vi "CSM Example - Caller is NOT a CSM.vi"() -> ()   [LabVIEW 2017]
uses:
  user.lib/_NEVSTOP/Communicable State Machine(CSM)/_Support/Common/Format Timestamp.vi
  user.lib/_NEVSTOP/Communicable State Machine(CSM)/Communicable State Machine.lvlib
  1. Create a reuse Module/1. Create a reuse Module.lvlib
panel:
  in  "UI: Front Panel State >> Close":bool
  in  "UI: Front Panel State >> Open":bool
  in  "API: Get Level":bool
  in  "Selected Module":string(combo)="SubModule0"
  in  "Level":dbl min=0.0 max=1.0 step=0.1
  out "Status History":string
  in  "API: Stop":bool
  in  "API: Start":bool
  in  "Unregister Status Change":bool
  in  "Register Status Change":bool
  out "error":errorcluster
  in  "Stop Module":bool
  in  "Start Module":bool
  out "Exist?":bool
  # "#CSM-Example Overview\n\n1. The purpose of this example is to demonstrate how to invoke the CSM module from other framework application. In this scenario, inter-module communication solely relies on Post/Send Message API and module status change user event. \n\nThis example asynchronously calls two instances of \"CSM Reuse Module.vi\", providing dynamic subscription to messages and manipulation of the underlying Module through the API."
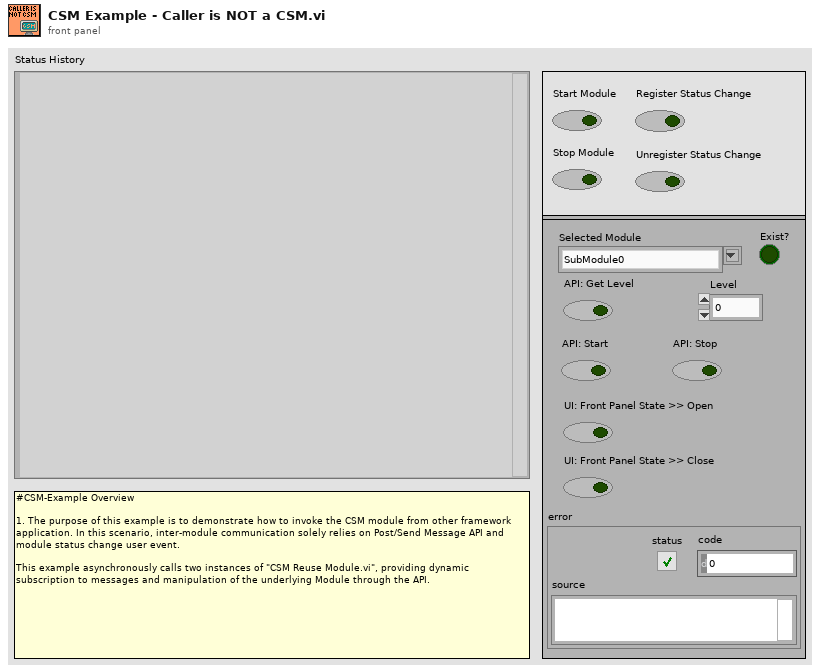
[diagram p1: front panel]
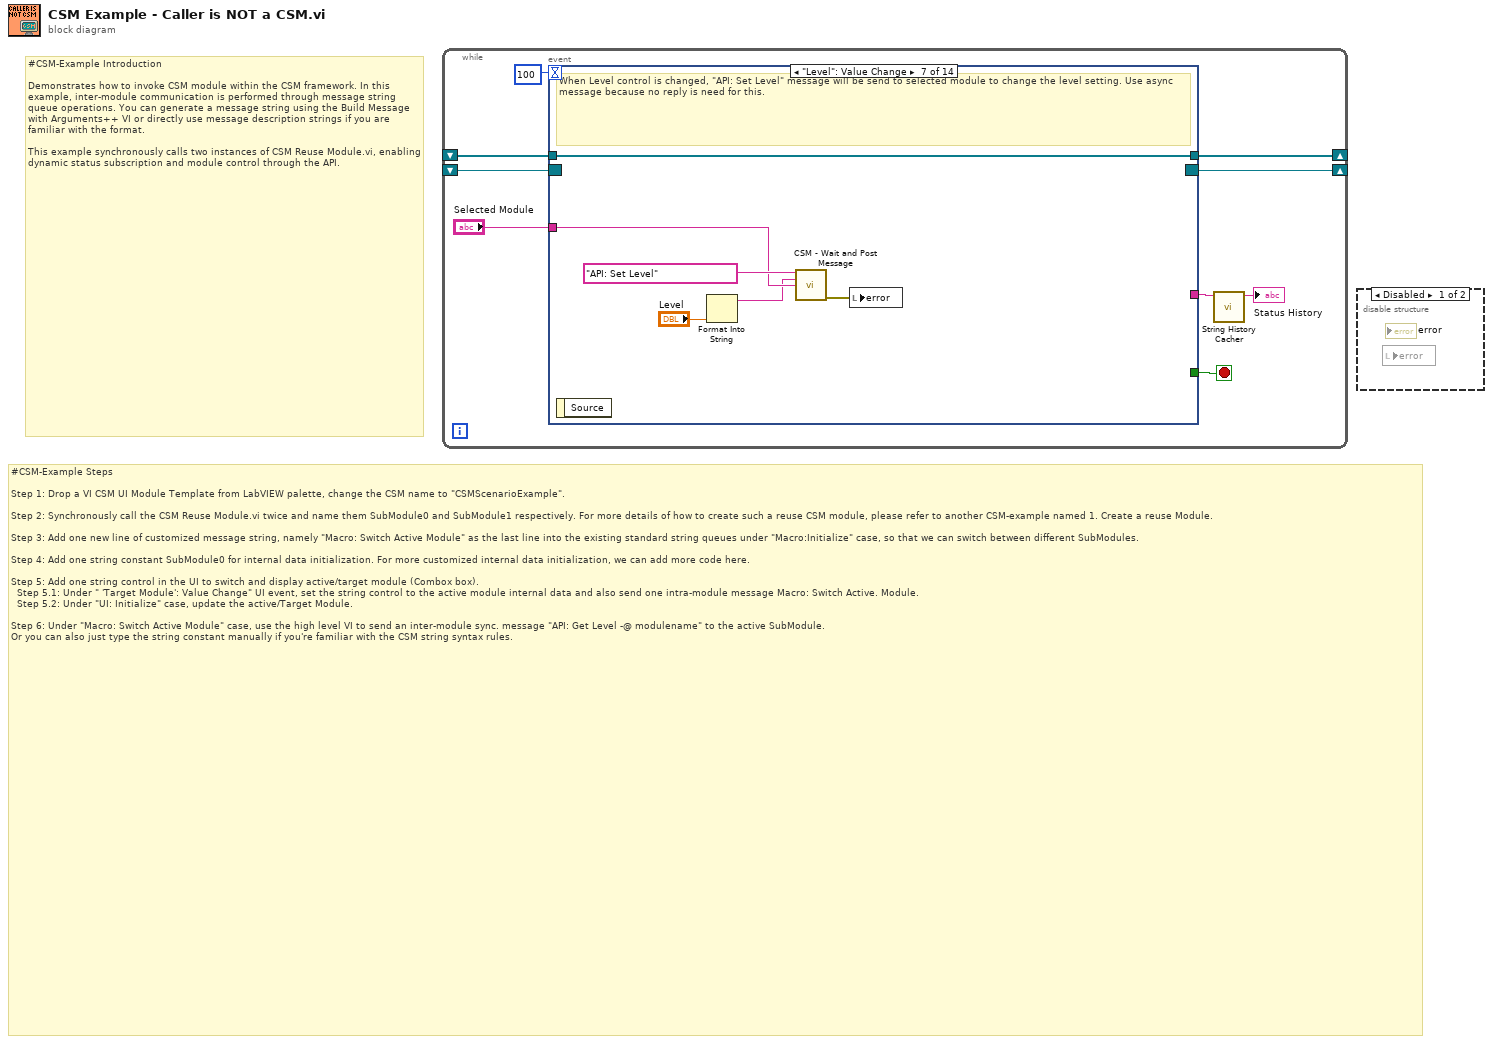
[diagram p0: block diagram]
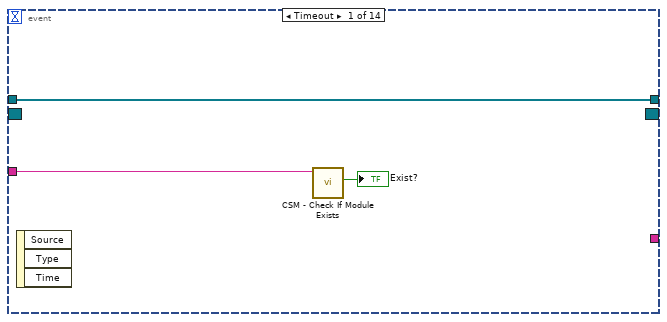
[diagram p3: hidden frame]
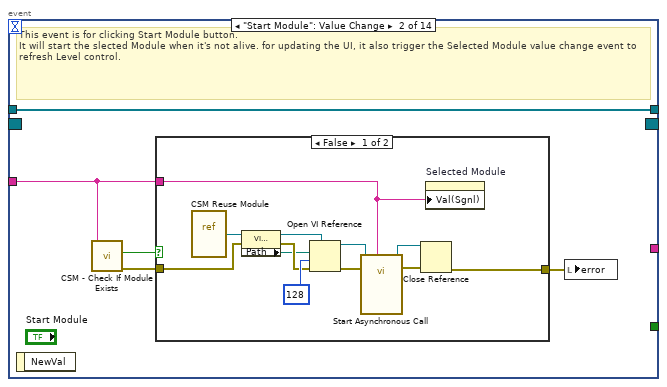
[diagram p4: hidden frame]
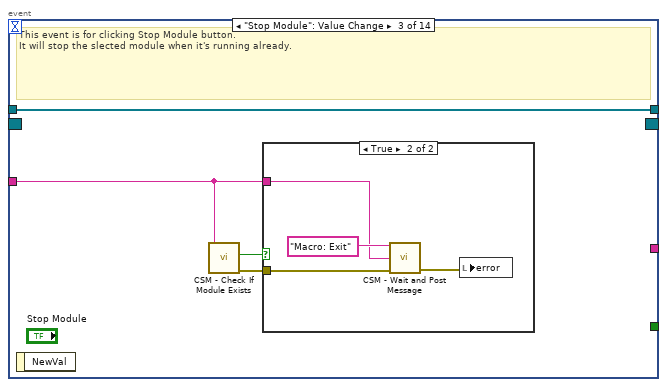
[diagram p6: hidden frame]
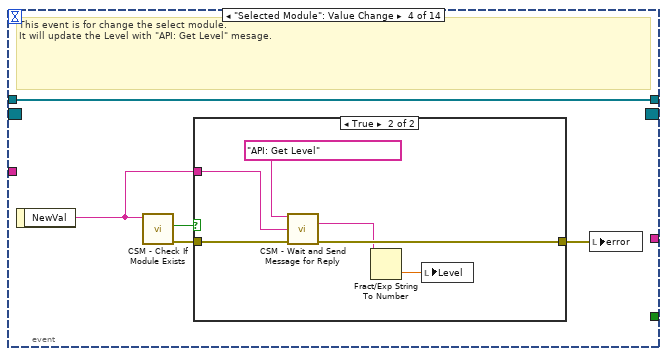
[diagram p8: hidden frame]
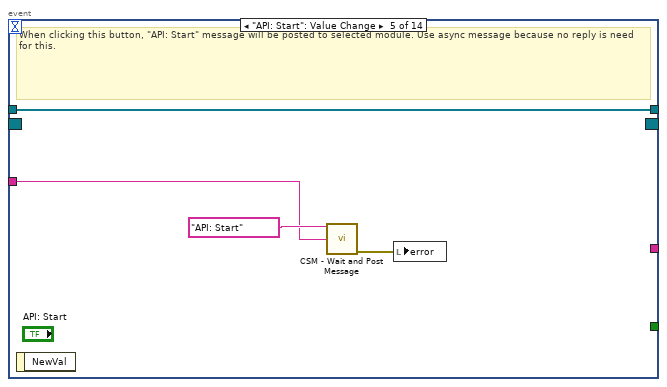
[diagram p10: hidden frame]
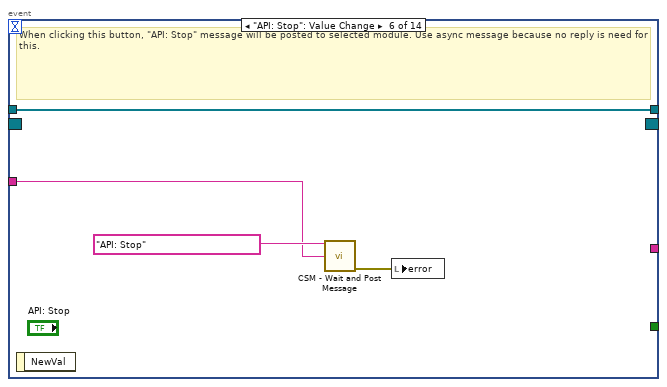
[diagram p11: hidden frame]
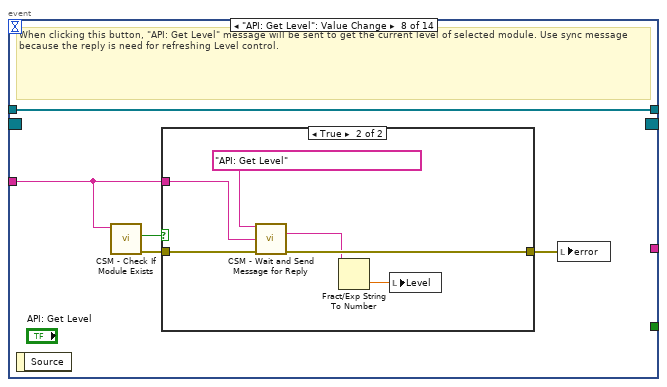
[diagram p12: hidden frame]
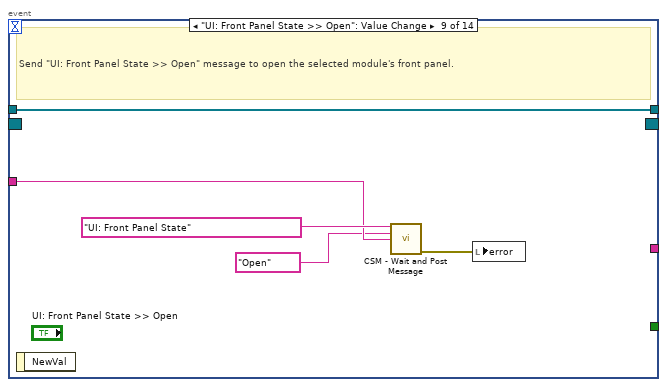
[diagram p14: hidden frame]
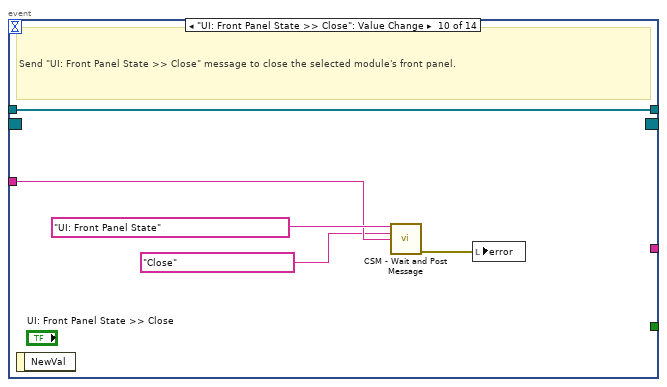
[diagram p15: hidden frame]
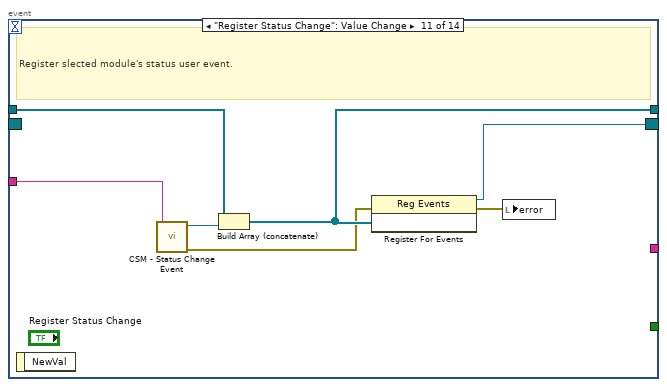
[diagram p16: hidden frame]
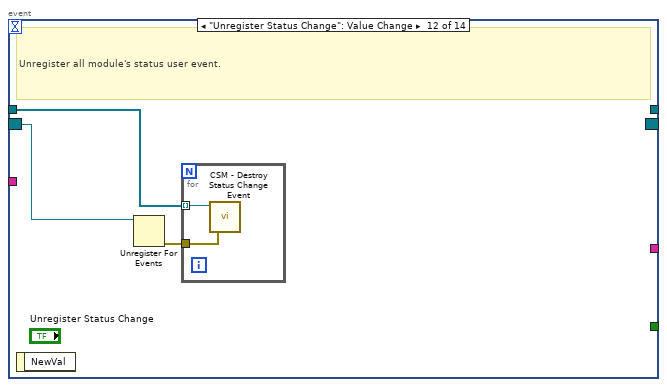
[diagram p17: hidden frame]
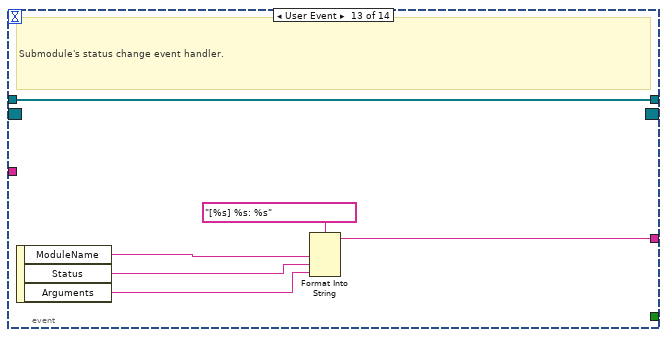
[diagram p18: hidden frame]
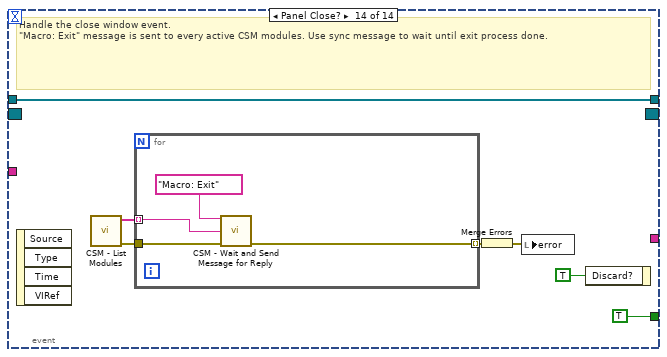
[diagram p19: hidden frame]
diagram:
  # "#CSM-Example Steps\n\nStep 1: Drop a VI CSM UI Module Template from LabVIEW palette, change the CSM name to \"CSMScenarioExample\".\n\nStep 2: Synchronously call the CSM Reuse Module.vi twice and name them SubModule0 and SubModule1 respectively. For more details of how to create such a reuse CSM module, please refer to another CSM-example named 1. Create a reuse Module.\n\nStep 3: Add one new line of customized message string, namely \"Macro: Switch Active Module\" as the last line into the existing standard string queues under \"Macro:Initialize\" case, so that we can switch between different SubModules.\n\nStep 4: Add one string constant SubModule0 for internal data initialization. For more customized internal data initialization, we can add more code here. \n\nStep 5: Add one string control in the UI to switch and display active/target module (Combox box).\n  Step 5.1: Under \" 'Target Module': Value Change\" UI event, set the string control to the active module internal data and also send one intra-module message Macro: Switch Active. Module. \n  Step 5.2: Under \"UI: Initialize\" case, update the active/Target Module.\n\nStep 6: Under \"Macro: Switch Active Module\" case, use the high level VI to send an inter-module sync. message \"API: Get Level -@ modulename\" to the active SubModule.\nOr you can also just type the string constant manually if you're familiar with the CSM string syntax rules."
  # "#CSM-Example Introduction\n\nDemonstrates how to invoke CSM module within the CSM framework. In this example, inter-module communication is performed through message string queue operations. You can generate a message string using the Build Message with Arguments++ VI or directly use message description strings if you are familiar with the format.\n\nThis example synchronously calls two instances of CSM Reuse Module.vi, enabling dynamic status subscription and module control through the API."
  n1 = while {
    shift-right: [w7] -> _
    shift-left: _ -> [w6]
    shift-right: [w5] -> _
    shift-left: _ -> [w4]
    stop <- w9 stop-if-true
    n2 = event shown="[6] \"Level\": Value Change" {
      selector: w6 -> [_ _ _ _ _ _ _ _ _ _ _ w96 _ _]
      dyn-events: [_ _ _ _ _ _ _ _ _ _ w93 _ _ _] -> w7
      timeout: 100 -> [_ _ _ _ _ _ _ _ _ _ _ _ _ _]
      tunnel: [_ _ _ _ _ _ _ _ _ _ _ _ _ TRUE ("Discard?")] -> w9
      tunnel: [w12 w17 w34 w42 w52 w56 w62 w68 w79 w84 w92 _ w99 w109] -> w5
      tunnel: w4 -> [w12 w17 w34 w42 w52 w56 w62 w68 w79 w84 w90 w94 w99 w109]
      tunnel: [_ _ _ _ _ _ _ _ _ _ _ _ w100 _] -> w2
      tunnel: "Selected Module" -> [w10 w13 w31 _ w51 w55 w61 w67 w78 w83 w89 _ _ _]
      event Timeout {
        n3 = event-data() -> ()  [unwired: 1 in, 3 out]
        n4 = call "CSM - Check If Module Exists.vi"("CSM Name"=w10) -> ("Exist?"=→"Exist?":bool)  [unwired: 8 in, 2 out]
      }
      event "Start Module": Value Change {
        # "This event is for clicking Start Module button. \nIt will start the slected Module when it's not alive. for updating the UI, it also trigger the Selected Module value change event to refresh Level control."
        n5 = event-data() -> ()  [unwired: 1 in, 1 out]
        n6 = call "CSM - Check If Module Exists.vi"("CSM Name"=w13) -> ("error out"=w15:errorcluster, "Exist?"=w16:bool)  [unwired: 8 in, 1 out]
        n7 = case shown="False" w16 {
          tunnel: w15 -> [w20 w30]
          tunnel: [w19 w30] -> w14
          tunnel: w13 -> [w18 _]
          frame False {
            n8 = vi-ref "CSM Reuse Module.vi"() -> (w22:refnum<vi>)
            n9 = property class="VI (strict)"(reference=w22, error in=w20) -> (reference out=w26:refnum<vi>, error out=w24:errorcluster, "Path"=w23:path)
            n10 = Open VI Reference(type specifier VI Refnum (for type only)=w26, vi path=w23, options=128, error in (no error)=w24) -> (vi reference=w25:refnum<vi>, error out=w21:errorcluster)  [unwired: 2 in]
            n11 = call-by-ref "Start Asynchronous Call"(reference=w25, error in=w21, "Name(\"\" to use uuid)"=w18) -> (reference out=w28:refnum<vi>, error out=w27:errorcluster)  [unwired: 11 in]
            n12 = Close Reference(reference=w28, error in (no error)=w27) -> (error out=w19:errorcluster)
            n13 = property on="Selected Module" class="CmbBox"("Val(Sgnl)"=w18) -> ()  [unwired: 2 in, 2 out]
          }
          frame True {
          }
        }
        n14 = local write "error"(w14) -> ()
      }
      event "Stop Module": Value Change {
        # "This event is for clicking Stop Module button. \nIt will stop the slected module when it's running already."
        n15 = event-data() -> ()  [unwired: 1 in, 1 out]
        n16 = call "CSM - Check If Module Exists.vi"("CSM Name"=w31) -> ("error out"=w32:errorcluster, "Exist?"=w33:bool)  [unwired: 8 in, 1 out]
        n17 = case shown="True" w33 {
          tunnel: w32 -> [_ w36]
          tunnel: w31 -> [_ w35]
          frame False {
          }
          frame True {
            n18 = call "CSM - Wait and Post Message.vi"("State"="Macro: Exit" ("States"), "Target Module"=w35, "Error In (No Error)"=w36) -> ("error out"=w37:errorcluster)  [unwired: 12 in]
            n19 = local write "error"(w37) -> ()
          }
        }
      }
      event "Selected Module": Value Change {
        # "This event is for change the select module.\nIt will update the Level with \"API: Get Level\" mesage."
        n20 = event-data() -> ("NewVal"=w39:string)  [unwired: 1 in]
        n21 = call "CSM - Check If Module Exists.vi"("CSM Name"=w39) -> ("error out"=w41:errorcluster, "Exist?"=w40:bool)  [unwired: 8 in, 1 out]
        n22 = case shown="True" w40 {
          tunnel: [w44 w49] -> w43
          tunnel: w39 -> [_ w46]
          tunnel: w41 -> [w44 w45]
          frame False {
          }
          frame True {
            n23 = call "CSM - Wait and Send Message for Reply.vi"("State"="API: Get Level", "Target Module"=w46, "Error In (No Error)"=w45) -> ("Response"=w47:string, "error out"=w49:errorcluster)  [unwired: 10 in, 1 out]
            n24 = Fract/Exp String To Number(string=w47) -> (number=w48:dbl)  [unwired: 3 in, 1 out]
            n25 = local write "Level"(w48) -> ()
          }
        }
        n26 = local write "error"(w43) -> ()
      }
      event "API: Start": Value Change {
        # "When clicking this button, \"API: Start\" message will be posted to selected module. Use async message because no reply is need for this."
        n27 = event-data() -> ()  [unwired: 1 in, 1 out]
        n28 = call "CSM - Wait and Post Message.vi"("State"="API: Start", "Target Module"=w51) -> ("error out"=w53:errorcluster)  [unwired: 13 in]
        n29 = local write "error"(w53) -> ()
      }
      event "API: Stop": Value Change {
        # "When clicking this button, \"API: Stop\" message will be posted to selected module. Use async message because no reply is need for this."
        n30 = event-data() -> ()  [unwired: 1 in, 1 out]
        n31 = call "CSM - Wait and Post Message.vi"("State"="API: Stop", "Target Module"=w55) -> ("error out"=w57:errorcluster)  [unwired: 13 in]
        n32 = local write "error"(w57) -> ()
      }
      event "Level": Value Change {
        # "When Level control is changed, \"API: Set Level\" message will be send to selected module to change the level setting. Use async message because no reply is need for this."
        n33 = event-data() -> ()  [unwired: 1 in, 1 out]
        n34 = Format Into String("Level") -> (resulting string=w59:string)  [unwired: 3 in, 1 out]
        n35 = call "CSM - Wait and Post Message.vi"("State"="API: Set Level", "Arguments (\"\")"=w59, "Target Module"=w61) -> ("error out"=w63:errorcluster)  [unwired: 12 in]
        n36 = local write "error"(w63) -> ()
      }
      event "API: Get Level": Value Change {
        # "When clicking this button, \"API: Get Level\" message will be sent to get the current level of selected module. Use sync message because the reply is need for refreshing Level control."
        n37 = event-data() -> ()  [unwired: 1 in, 1 out]
        n38 = call "CSM - Check If Module Exists.vi"("CSM Name"=w67) -> ("error out"=w66:errorcluster, "Exist?"=w65:bool)  [unwired: 8 in, 1 out]
        n39 = case shown="True" w65 {
          tunnel: [w70 w75] -> w69
          tunnel: w67 -> [_ w72]
          tunnel: w66 -> [w70 w71]
          frame False {
          }
          frame True {
            n40 = call "CSM - Wait and Send Message for Reply.vi"("State"="API: Get Level", "Target Module"=w72, "Error In (No Error)"=w71) -> ("Response"=w73:string, "error out"=w75:errorcluster)  [unwired: 10 in, 1 out]
            n41 = Fract/Exp String To Number(string=w73) -> (number=w74:dbl)  [unwired: 3 in, 1 out]
            n42 = local write "Level"(w74) -> ()
          }
        }
        n43 = local write "error"(w69) -> ()
      }
      event "UI: Front Panel State >> Open": Value Change {
        # "Send \"UI: Front Panel State >> Open\" message to open the selected module's front panel."
        n44 = event-data() -> ()  [unwired: 1 in, 1 out]
        n45 = call "CSM - Wait and Post Message.vi"("State"="UI: Front Panel State", "Arguments (\"\")"="Open" ("Arguments (\"\")"), "Target Module"=w78) -> ("error out"=w80:errorcluster)  [unwired: 12 in]
        n46 = local write "error"(w80) -> ()
      }
      event "UI: Front Panel State >> Close": Value Change {
        # "Send \"UI: Front Panel State >> Close\" message to close the selected module's front panel."
        n47 = event-data() -> ()  [unwired: 1 in, 1 out]
        n48 = call "CSM - Wait and Post Message.vi"("State"="UI: Front Panel State", "Arguments (\"\")"="Close" ("Arguments (\"\")"), "Target Module"=w83) -> ("error out"=w85:errorcluster)  [unwired: 12 in]
        n49 = local write "error"(w85) -> ()
      }
      event "Register Status Change": Value Change {
        # "Register slected module's status user event."
        n50 = event-data() -> ()  [unwired: 1 in, 1 out]
        n51 = call "CSM - Status Change Event.vi"("CSM Module"=w89) -> ("error out"=w88:errorcluster, "Status Change Event"=w91:refnum<user-event>)  [unwired: 8 in, 1 out]
        n52 = Build Array (concatenate)(w90, w91) -> (w92:refnum<user-event>[])
        n53 = register-events(error in=w88, w92) -> (reference out=w93:refnum<event-registration>, error out=w87:errorcluster)  [unwired: 1 in]
        n54 = local write "error"(w87) -> ()
      }
      event "Unregister Status Change": Value Change {
        # "Unregister all module's status user event."
        n55 = event-data() -> ()  [unwired: 1 in, 1 out]
        n56 = Unregister For Events(event registration refnum=w96) -> (error out=w95:errorcluster)  [unwired: 1 in]
        n57 = for {
          tunnel: w95 -> [w98]
          tunnel: w94 -> [w97] mode=indexing
          n58 = call "CSM - Destroy Status Change Event.vi"("Error In"=w98, "Status Change Event"=w97) -> ()  [unwired: 9 in, 1 out]
        }
      }
      event User Event {
        # "Submodule's status change event handler."
        n59 = event-data() -> ("ModuleName"=w104:string, "Status"=w103:string, "Arguments"=w102:string)  [unwired: 1 in]
        n60 = Format Into String(format string="[%s] %s: %s", w104, w103, w102) -> (resulting string=w100:string)  [unwired: 2 in, 1 out]
      }
      event Panel Close? {
        # "Handle the close window event. \n\"Macro: Exit\" message is sent to every active CSM modules. Use sync message to wait until exit process done."
        n61 = event-data() -> ()  [unwired: 1 in, 4 out]
        n62 = call "CSM - List Modules.vi"() -> ("error out"=w106:errorcluster, "Module Names"=w105:string[])  [unwired: 10 in]
        n63 = for {
          tunnel: [w114] -> w108 mode=indexing
          tunnel: w106 -> [w113]
          tunnel: w105 -> [w112] mode=indexing
          n64 = call "CSM - Wait and Send Message for Reply.vi"("State"="Macro: Exit" ("States"), "Target Module"=w112, "Error In (No Error)"=w113) -> ("error out"=w114:errorcluster)  [unwired: 10 in, 2 out]
        }
        n65 = Merge Errors(w108) -> (w107:errorcluster)
        n66 = local write "error"(w107) -> ()
        n67 = event-data("Discard?"=TRUE) -> ()  [unwired: 1 in, 1 out]
      }
    }
    n68 = call "String History Cacher.vi"("String"=w2) -> ("String Cache"=→"Status History":string)  [unwired: 10 in]
  }
  n69 = disable-structure shown="Disabled" {
    frame Disabled {
      n70 = local read "error"() -> ()  [unwired: 1 in]
    }
    frame Enabled {
    }
  }
